vi "Dequeue Message.vi"(8 "Error In":errorcluster, 10 "timeout in ms (-1)":i32=-1, 11 "Message Queue":refnum<queue>) -> (0 "Error Out":errorcluster, 1 "Message Data":variant, 2 "Message":string, 3 "dup Message Queue":refnum<queue>, 4 "timed out?":bool)   [LabVIEW 2020]
doc: "This VI pulls messages off the Message Queue. It has special error handling to account for an error occurring on the last iteration of the Message Handling Loop.\n\nNo Error - normal Dequeue Element operation.\nError - check if it is an error code we wish to ignore. If so, clear the error and perform a normal Dequeue Element. If not, output the error, and put a 'Stop' message on the Message Queue."
uses:
  Typedefs/Message Cluster.ctl
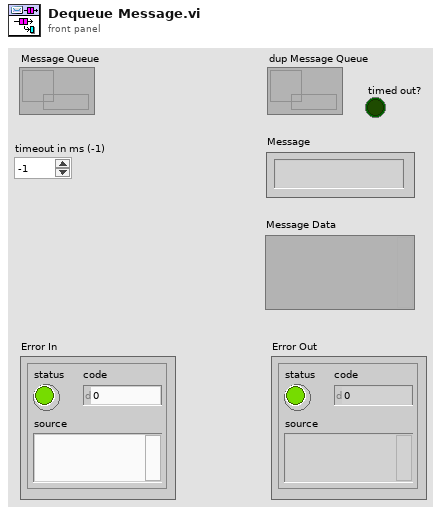
[diagram p1: front panel]
types:
  T1 = typedef "Message Cluster.ctl" = cluster{"Message":string, "Message Data":variant}
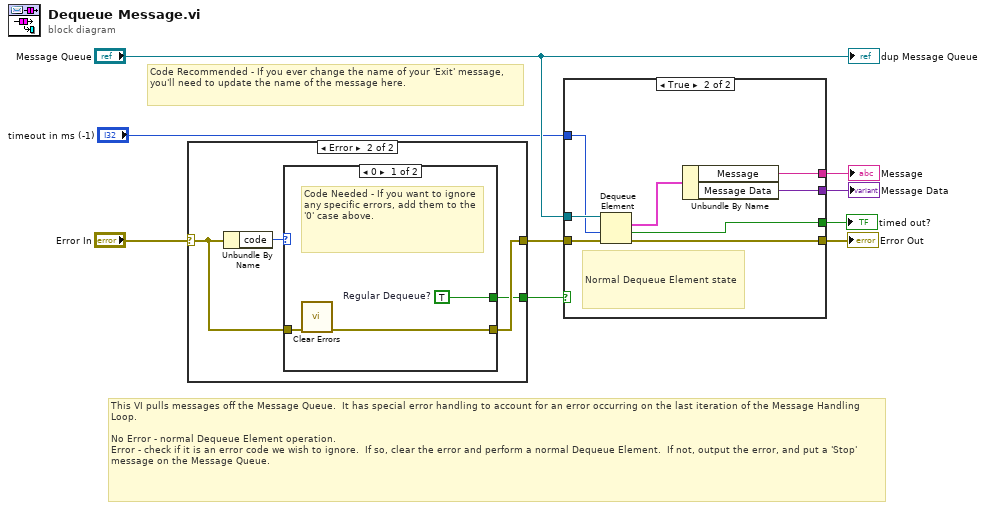
[diagram p0: block diagram]
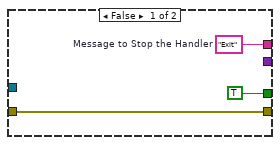
[diagram p2: hidden frame]
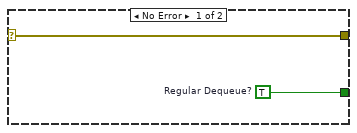
[diagram p3: hidden frame]
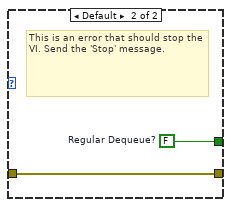
[diagram p4: hidden frame]
diagram:
  # "Code Recommended - If you ever change the name of your 'Exit' message, you'll need to update the name of the message here."
  # "This VI pulls messages off the Message Queue.  It has special error handling to account for an error occurring on the last iteration of the Message Handling Loop.\n\nNo Error - normal Dequeue Element operation.\nError - check if it is an error code we wish to ignore.  If so, clear the error and perform a normal Dequeue Element.  If not, output the error, and put a 'Stop' message on the Message Queue."
  n1 = case shown="Error" "Error In" {
    selector: "Error In" -> [w11 w14]
    tunnel: [w11 w13] -> w9
    tunnel: [w10 w12] -> w8
    frame No Error {
      w10 = TRUE  # Regular Dequeue?
    }
    frame Error {
      n2 = Unbundle By Name(w14) -> ("code"=w15:i32)
      n3 = case shown="0" w15 {
        tunnel: [w18 w20] -> w13
        tunnel: w14 -> [w17 w20]
        tunnel: [w16 w19] -> w12
        frame 0 {
          w16 = TRUE  # Regular Dequeue?
          # "Code Needed - If you want to ignore any specific errors, add them to the '0' case above."
          n4 = call <vilib>:"Clear Errors.vi"("error in (no error)"=w17) -> ("error out"=w18:errorcluster)  [unwired: 5 in, 1 out]
        }
        frame Default {
          w19 = FALSE  # Regular Dequeue?
          # "This is an error that should stop the VI. Send the 'Stop' message."
        }
      }
    }
  }
  n5 = case shown="True" w8 {
    tunnel: [w23 w31] -> w3
    tunnel: w9 -> [w23 w30]
    tunnel: "Message Queue" -> [_ w29]
    tunnel: [w22 w27] -> w6
    tunnel: [_ w26] -> w5
    tunnel: "timeout in ms (-1)" -> [_ w25]
    tunnel: [TRUE ("timed out?") w24] -> w1
    frame False {
      w22 = "Exit"  # Message to Stop the Handler
    }
    frame True {
      # "Normal Dequeue Element state"
      n6 = Dequeue Element(queue=w29, timeout in ms (-1)=w25, error in (no error)=w30) -> (element=w28:T1, timed out?=w24:bool, error out=w31:errorcluster)  [unwired: 1 out]
      n7 = Unbundle By Name(w28) -> ("Message"=w27:string, "Message Data"=w26:variant)
    }
  }
  "Message" <- w6
  "Message Data" <- w5
  "Error Out" <- w3
  "timed out?" <- w1
  "dup Message Queue" <- "Message Queue"
